vi "Component UI Test.vi"() -> ()   [LabVIEW 2017, in "DSF Core.lvlib"]
uses:
  DSF Core.lvlib
  Classes/Component User Interface/UI Type.ctl
  Classes/User Interface/Core/Core User Interfaces.lvclass
  Components/Transceivers/UDP/Configuration/UDP Configurations.lvclass
  C:/Git/DSF/Core/Classes/Component Configuration/Component Configurations.lvclass
  Components/Transceivers/UDP/UI/UDP User Interfaces.lvclass
  Typedefs/DSF Settings Info.ctl
  Typedefs/DSF Version Info.ctl
  Classes/Configuration/Core/Core Configurations.lvclass
  Classes/User Interface/Settings Editor/Settings Editor.lvclass
  C:/Git/DSF/Core/Classes/User Interface/User Interface.lvclass
  Classes/User Interface/User Interface.lvclass
  Classes/Configuration/Configuration.lvclass
  Classes/Component/Component.lvclass
  Classes/User Interface Handler/User Interface Handler.lvclass
  Classes/Component Configuration/Component Configurations.lvclass
  Classes/Component User Interface/Component User Interfaces.lvclass
panel:
  in  "UI Type":T1=enum."Thread"
  in  "stop":bool
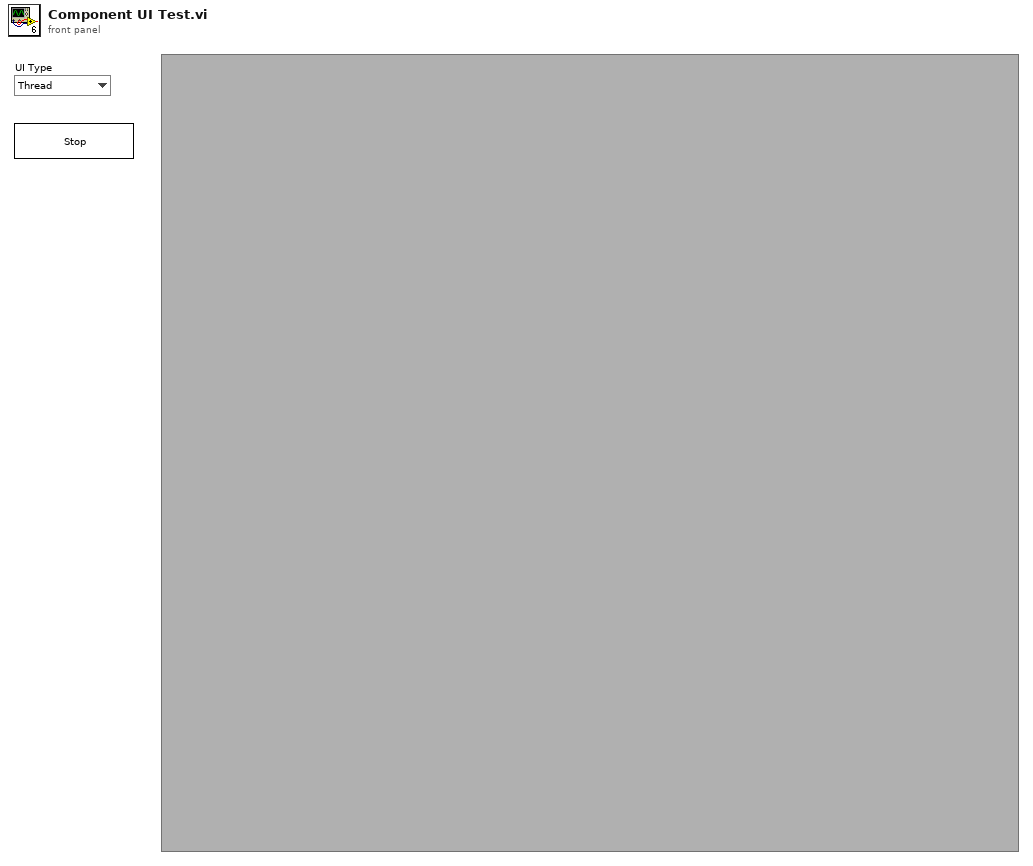
[diagram p1: front panel]
types:
  T1 = typedef "DSF Core.lvlib/Component User Interfaces.lvclass/UI Type.ctl" = enum16{"Plugin", "Thread", "Rx Group", "Tx Group", "Rx Transfer", "Tx Transfer", "Rx Channel", "Tx Channel"}
  T2 = typedef "DSF Core.lvlib/DSF Settings Info.ctl" = cluster{"component":string, "version":T3, "values":cluster{"key":string, "value":string}[]}
  T3 = typedef "DSF Core.lvlib/DSF Version Info.ctl" = cluster{"major":u32, "minor":u32, "fix":u32, "build":string}
  T4 = typedef "DSF Core.lvlib/User Interface Handler.lvclass/User Interface Ref.ctl" = refnum<vi>
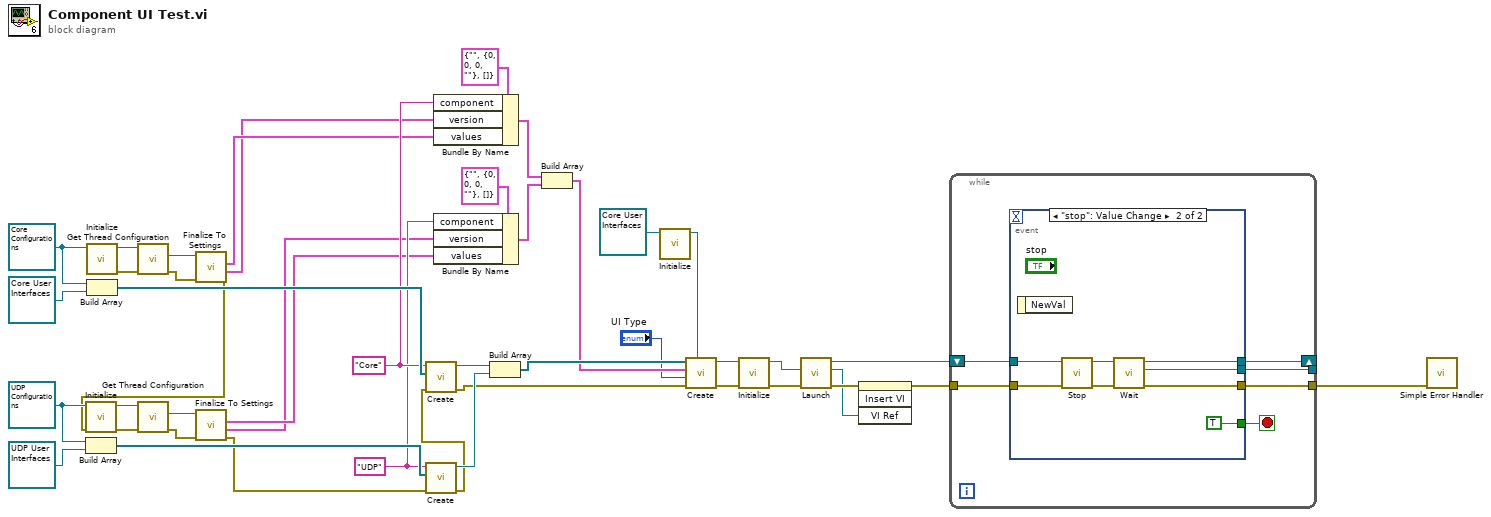
[diagram p0: block diagram]
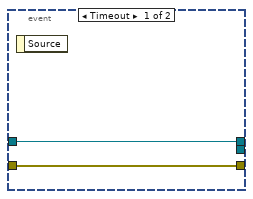
[diagram p2: hidden frame]
diagram:
  w30 = refnum<class "Core Configurations.lvclass"> refnum ("DSF Core.lvlib:Core Configurations.lvclass")
  w27 = refnum<class "UDP Configurations.lvclass"> refnum ("DSF Core.lvlib:UDP Configurations.lvclass")
  w28 = "UDP" ("name")
  w31 = "Core" ("name")
  n1 = Build Array(w27, refnum<class "UDP User Interfaces.lvclass"> refnum ("DSF Core.lvlib:UDP Configuration User Interfaces.lvclass")) -> (w38:refnum<class>[])
  n2 = call-dynamic "Initialize.vi"("Core Configuration in"=w30) -> ("error out"=w17:errorcluster, "Core Configuration out"=w29:refnum<class "Core Configurations.lvclass">)  [unwired: 9 in]
  n3 = Build Array(w30, refnum<class "Core User Interfaces.lvclass"> refnum ("DSF Core.lvlib:Core Configuration UI.lvclass")) -> (w39:refnum<class>[])
  n4 = call "Get Thread Configuration.vi"("error in (no error)"=w17, "Component Configuration in"=w29) -> ("error out"=w16:errorcluster, "Thread Configuration"=w23:refnum<class "Configuration.lvclass">)  [unwired: 7 in, 1 out]
  n5 = call-dynamic "Finalize To Settings.vi"("error in (no error)"=w16, "Configuration in"=w23) -> ("error out"=w15:errorcluster, "settings version"=w18:T3, "settings"=w22:cluster{"key":string, "value":string}[])  [unwired: 6 in, 1 out]
  n6 = call-dynamic "Initialize.vi"("error in (no error)"=w15, "UDP Configuration in"=w27) -> ("error out"=w14:errorcluster, "UDP Configuration out"=w26:refnum<class "UDP Configurations.lvclass">)  [unwired: 8 in]
  n7 = call "Get Thread Configuration.vi"("error in (no error)"=w14, "Component Configuration in"=w26) -> ("error out"=w13:errorcluster, "Thread Configuration"=w21:refnum<class "Configuration.lvclass">)  [unwired: 7 in, 1 out]
  n8 = call-dynamic "Finalize To Settings.vi"("error in (no error)"=w13, "Configuration in"=w21) -> ("error out"=w12:errorcluster, "settings version"=w19:T3, "settings"=w20:cluster{"key":string, "value":string}[])  [unwired: 6 in, 1 out]
  n9 = call "Create.vi"("error in (no error)"=w12, "objects"=w38, "name"=w28) -> ("error out"=w11:errorcluster, "Component"=w44:refnum<class "Component.lvclass">)  [unwired: 7 in]
  n10 = call "Create.vi"("error in (no error)"=w11, "objects"=w39, "name"=w31) -> ("error out"=w8:errorcluster, "Component"=w43:refnum<class "Component.lvclass">)  [unwired: 7 in]
  n11 = Bundle By Name(cluster=T2 {"component"="", "version"={"major"=0, "minor"=0, "fix"=0, "build"=""}, "values"=[]} ("component settings"), "component"=w31, "version"=w18, "values"=w22) -> (w25:T2)
  n12 = Bundle By Name(cluster=T2 {"component"="", "version"={"major"=0, "minor"=0, "fix"=0, "build"=""}, "values"=[]} ("component settings"), "component"=w28, "version"=w19, "values"=w20) -> (w24:T2)
  n13 = Build Array(w43, w44) -> (w7:refnum<class "Component.lvclass">[])
  n14 = Build Array(w25, w24) -> (w6:T2[])
  n15 = call-dynamic "Initialize.vi"("Component UI in"=refnum<class "Core User Interfaces.lvclass"> refnum ("Core User Interfaces")) -> ("Component UI out"=w3:refnum<class "Core User Interfaces.lvclass">)  [unwired: 9 in, 1 out]
  n16 = call "Create.vi"("Core User Interfaces"=w3, "error in (no error)"=w8, "user interface type"="UI Type", "component settings"=w6, "Components"=w7) -> ("error out"=w10:errorcluster, "Settings Editor out"=w9:refnum<class "Settings Editor.lvclass">)  [unwired: 5 in]
  n17 = call-dynamic "Initialize.vi"("error in (no error)"=w10, "Settings Editor in"=w9) -> ("error out"=w37:errorcluster, "Settings Editor out"=w36:refnum<class "Settings Editor.lvclass">)  [unwired: 8 in]
  n18 = call "Launch.vi"("error in (no error)"=w37, "User Interface"=w36) -> ("error out"=w42:errorcluster, "active vi"=w40:T4, "User Interface Handler out"=w35:refnum<class "User Interface Handler.lvclass">)  [unwired: 7 in]
  n19 = invoke on="Sub Panel" class="SubPnl" method="Insert VI"(error in=w42, "VI Ref"=w40) -> (error out=w41:errorcluster)  [unwired: 2 in, 3 out]
  n20 = while {
    tunnel: w41 -> [w49]
    tunnel: [w48] -> w34
    shift-right: [w46] -> _
    shift-left: w35 -> [w47]
    tunnel: [w45] -> _
    stop <- w50 stop-if-true
    n21 = event shown="[1] \"stop\": Value Change" {
      selector: _ -> [_ _]
      dyn-events: _ -> [_ _]
      timeout: _ -> [_ _]
      tunnel: [_ TRUE] -> w50
      tunnel: w49 -> [w51 w58]
      tunnel: [w51 w55] -> w48
      tunnel: w47 -> [w52 w57]
      tunnel: [w52 w54] -> w46
      tunnel: [_ w53] -> w45
      event Timeout {
        n22 = event-data() -> ()  [unwired: 1 in, 1 out]
      }
      event "stop": Value Change {
        n23 = event-data() -> ()  [unwired: 1 in, 1 out]
        n24 = call "Stop.vi"("error in (no error)"=w58, "User Interface Handler in"=w57) -> ("error out"=w59:errorcluster, "User Interface Handler out"=w56:refnum<class "User Interface Handler.lvclass">)  [unwired: 8 in]
        n25 = call "Wait.vi"("error in (no error)"=w59, "User Interface Handler in"=w56) -> ("error out"=w55:errorcluster, "User Interface"=w53:refnum<class "User Interface.lvclass">, "User Interface Handler out"=w54:refnum<class "User Interface Handler.lvclass">)  [unwired: 7 in]
      }
    }
  }
  n26 = call <vilib>:"Simple Error Handler.vi"("error in (no error)"=w34) -> ()  [unwired: 4 in, 5 out]
